vi "nanostage-set.vi"(3 "error in":errorcluster, 4 "setValues":dbl[](array[numeric]), 5 "Axes to move":string[](array[string])) -> (0 "error out":errorcluster, 1 "moving":bool, 2 "getValues":cluster{"postion":dbl[], "status":bool[]})   [LabVIEW 2017]
panel:
  in  "wait for movement":bool=TRUE
  # "3D piezo nano stage"
  # "x-axis"
  # "y-axis"
  # "z-axis"
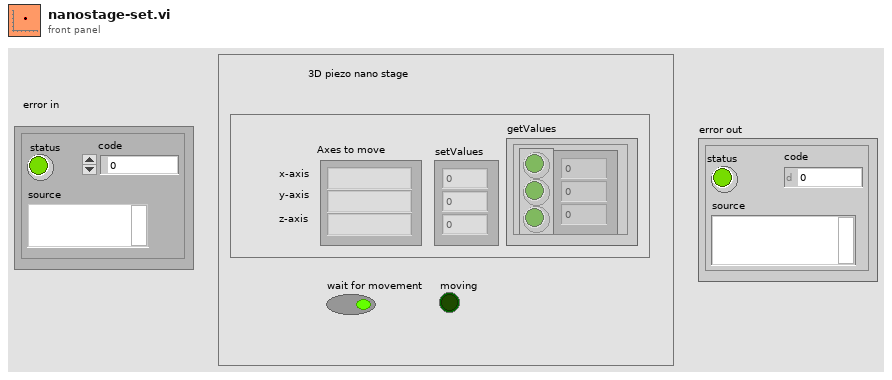
[diagram p1: front panel]
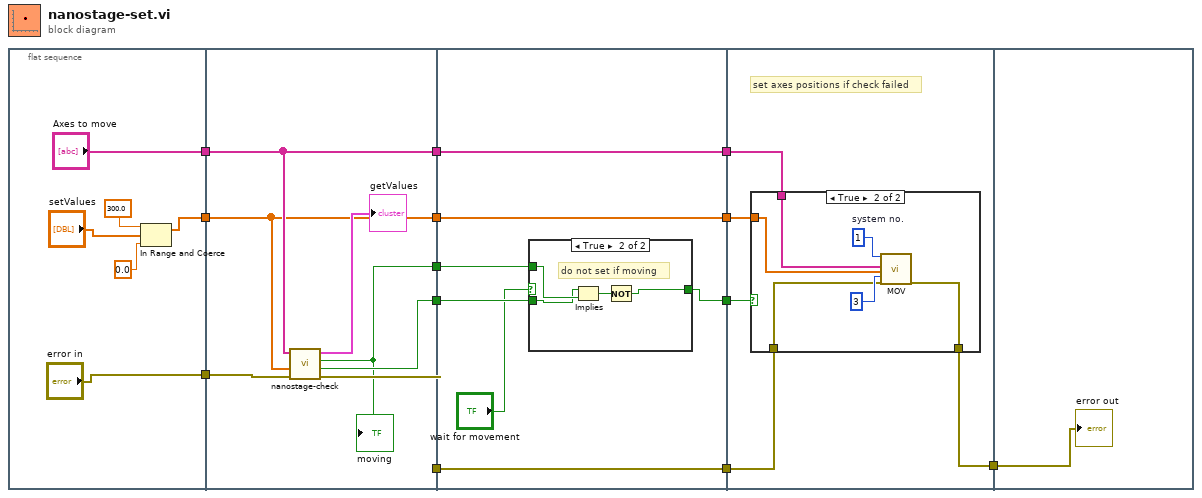
[diagram p0: block diagram]
diagram:
  n1 = flat-sequence {
    tunnel: ["error in"] -> w13
    tunnel: ["Axes to move"] -> w11
    tunnel: [w14] -> w1
    tunnel: [w23] -> w10
    tunnel: [w26] -> w8
    tunnel: [w20] -> w6
    tunnel: w13 -> [w24]
    tunnel: w11 -> [w22]
    tunnel: [w22] -> w4
    tunnel: [w21] -> w2
    tunnel: w1 -> [w20]
    tunnel: w10 -> [w30]
    tunnel: [w29] -> w9
    tunnel: w8 -> [w33]
    tunnel: [w33] -> w7
    tunnel: w6 -> [w32]
    tunnel: [w32] -> w5
    tunnel: w4 -> [w31]
    tunnel: [w31] -> w3
    tunnel: w2 -> [w28]
    tunnel: w9 -> [w43]
    tunnel: w7 -> [w42]
    tunnel: w5 -> [w41]
    tunnel: [w40] -> w12
    tunnel: w3 -> [w39]
    tunnel: w12 -> [w51]
    frame #0 {
      n2 = In Range and Coerce(upper limit=300.0, x="setValues", lower limit=0.0) -> (coerced(x)=w14:dbl[])  [unwired: 1 out]
    }
    frame #1 {
      n3 = call "nanostage-check.vi"("error in"=w24, "axis set values"=w20, "Axes to move"=w22) -> ("error out"=w26:errorcluster, "parameters not ok"=w23:bool, "moving"=w21:bool, "get Values"=→"getValues":cluster{"postion":dbl[], "status":bool[]})  [unwired: 1 in]
      "moving" <- w21
    }
    frame #2 {
      n4 = case shown="True" "wait for movement" {
        selector: "wait for movement" -> [w34 _]
        tunnel: w30 -> [_ w37]
        tunnel: [w34 w35] -> w29
        tunnel: w28 -> [_ w38]
        frame False {
        }
        frame True {
          # "do not set if moving"
          n5 = Implies(1:w38, 2:w37) -> (0:w36:bool)
          n6 = Not(x=w36) -> (.not. x?=w35:bool)
        }
      }
    }
    frame #3 {
      # "set axes positions if check failed"
      n7 = case shown="True" w43 {
        tunnel: w42 -> [w44 w48]
        tunnel: [w44 w47] -> w40
        tunnel: w39 -> [_ w46]
        tunnel: w41 -> [_ w45]
        frame False {
        }
        frame True {
          w49 = 1  # system no.
          n8 = call "MOV.vi"("System no."=w49, "Axes to move"=w46, "Position values"=w45, "No.of digits"=i16 3, "error in"=w48) -> ("error out"=w47:errorcluster)  [unwired: 14 in]
        }
      }
    }
    frame #4 {
      "error out" <- w51
    }
  }
